vi "Get All Measured Values.vi"(0 "VISA Session In":refnum<visa-resource-name>="OXYMAT", 1 "Target Address":u8=16 format="%.0x", 2 "Source Address":u8=208 format="%.0x", 7 "Use Broadcast?(F)":bool, 11 "error in (no error)":errorcluster) -> (4 "VISA Session Out":refnum<visa-resource-name>, 6 "Message Header":T3 {"Source Address" format="%.0x"; "Target Address" format="%.0x"}, 8 "Measurements":cluster{"Measured value":dbl, "Dimension":T1}[](array[cluster]) {"Measured value" format="%#_6f"}, 10 "Measured variables":T2[](array[typedef]), 13 "Success":bool, 15 "error out":errorcluster)   [LabVIEW 2020, in "Siemens ELAN.lvlib"]
doc: "Using the Siemens ELAN protocol, gets all measured values from a channel. The input boolean 'Use Broadcast?' determines whether the values are actively requested, or whether this VI passively waits for a broadcast telegram. Returns array of measured real values and units of measure, plus a matching array of measured variable types. Also returns a boolean indicating that the addressed device provided a valid response.\n\n$Revision:: 0 $\n$Modtime:: yy-mm-dd hh:mm $\n$Author:: Dboyd $"
uses:
  Siemens ELAN.lvlib
  Unit Dimensions.ctl
  Measured variables.ctl
  Message Header.ctl
  Channel Status.ctl
panel:
  in  "Measured variable":T2
  in  "Dimension":T1
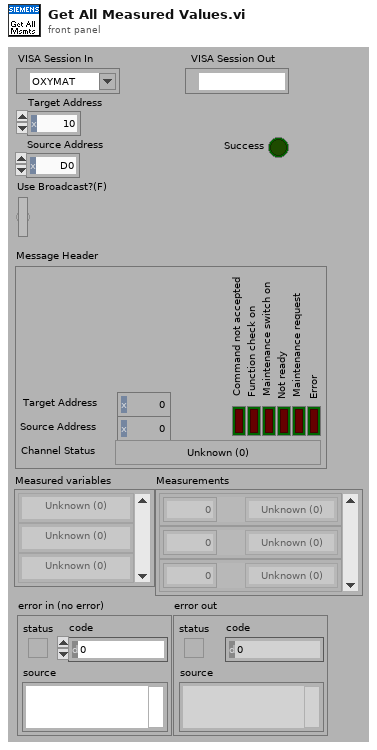
[diagram p1: front panel]
types:
  T1 = typedef "Siemens ELAN.lvlib/Unit Dimensions.ctl" = enum8{"Unknown (0)", "Pure number", "ppm", "ppb", "vpm", "vpm C1", "vpm C3", "vpm C6", "mg C/m^3", "mg/m^3", "%", "% v/v", "% of range", "% saturation", "%/°C", "%/K", "% w/w", "mV/pH", "mV/mbar", "nA/mbar", "S/m", "S/cm", "mS/m", "mS/cm", "uS/m", "uS/cm", "s", "min", "hr", "pA", "mA", "uV", "mV", "V", "mbar", "hPa", "ml/min", "kohm", "MOhm", "S", "°C", "Hz", "pH", "ug/l", "mg/l", "l/min", "uA", "mg/dm^3", "kPa", "kohm*cm", "MOhm*cm", "°", "Unknown (>51)"}
  T2 = typedef "Siemens ELAN.lvlib/Measured variables.ctl" = enum8{"Unknown (0)", "No component", "CO", "CO2", "CH4", "C6H14", "SO2", "NO", "NO2", "CHClF2 (R22)", "C3H8", "C4H10", "O2", "C5H12", "HC", "Pressure", "pH", "Temperature", "C2H4", "C2H2", "C3H6", "C4H6", "C4H8", "C2H6", "NH3", "N2O", "C6H6", "SF6", "CH3OH", "C2H5OH", "CH2Cl2", "C2H4Cl2", "CH3Cl", "C2H4O", "H2O (vapor)", "G/l", "Unknown (36)", "Unknown (37)", "Unknown (38)", "Unknown (39)", "Unknown (40)", "Unknown (41)", "Unknown (42)", "Unknown (43)", "Unknown (44)", "Unknown (45)", "Unknown (46)", "Unknown (47)", "Unknown (48)", "Unknown (49)", "Unknown (50)", "Unknown (51)", "Unknown (52)", "Unknown (53)", "Unknown (54)", "Unknown (55)", "Unknown (56)", "Unknown (57)", "Unknown (58)", "Unknown (59)", "Unknown (60)", "Unknown (61)", "Unknown (62)", "Unknown (63)", "Unknown (64)", "Unknown (65)", "Unknown (66)", "Unknown (67)", "Unknown (68)", "Unknown (69)", "Unknown (70)", "Unknown (71)", "Unknown (72)", "Unknown (73)", "Unknown (74)", "Unknown (75)", "Unknown (76)", "Unknown (77)", "Unknown (78)", "Unknown (79)", "Unknown (80)", "Unknown (81)", "Unknown (82)", "Unknown (83)", "Unknown (84)", "Unknown (85)", "Unknown (86)", "Unknown (87)", "Unknown (88)", "Unknown (89)", "Unknown (90)", "Unknown (91)", "Unknown (92)", "Unknown (93)", "Unknown (94)", "Unknown (95)", "Unknown ((96)", "Unknown (97)", "Unknown (98)", "Unknown (99)", "Ambient Pressure", "Unknown (>100)"}
  T3 = typedef "Siemens ELAN.lvlib/Message Header.ctl" = cluster{"Target Address":u8, "Source Address":u8, "Error":bool, "Maintenance request":bool, "Not ready":bool, "Maintenance switch on":bool, "Function check on":bool, "Command not accepted":bool, "Channel Status":T4}
  T4 = typedef "Siemens ELAN.lvlib/Channel Status.ctl" = enum8{"Unknown (0)", "Warm-up", "Pause", "Standby", "Measure", "Zero calibration", "Adjust component slope", "Unknown (7)", "Adjust curve dip", "Adjust linearization sensitivity", "Adjust temperature compensation", "Adjust pressure compensation", "Adjust linearization zero", "Adjust flow sensor", "Autocal", "Adjust phase", "Zero calibration of O2 sensor", "Synchronous zero calibration", "Purging for synchronous zero calibration", "Adjust analog output", "Adjust analog input", "Cleaning", "Unknown (>21)"}
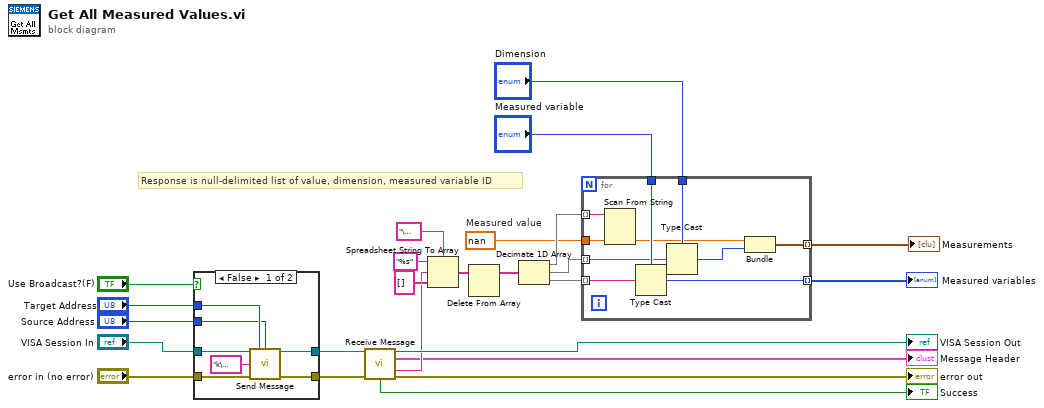
[diagram p0: block diagram]
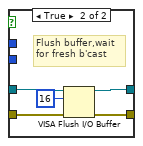
[diagram p2: hidden frame]
diagram:
  w5 = nan  # Measured value
  # "Response is null-delimited list of value, dimension, measured variable ID"
  n1 = case shown="False" "Use Broadcast?(F)" {
    tunnel: [w32 w36] -> w25
    tunnel: [w31 w34] -> w24
    tunnel: "VISA Session In" -> [w30 w37]
    tunnel: "error in (no error)" -> [w29 w35]
    tunnel: "Target Address" -> [w28 _]
    tunnel: "Source Address" -> [w27 _]
    frame False {
      n2 = call "Send Message.vi"("VISA Session In"=w30, "Target Address"=w28, "Source Address"=w27, "Command"="k\u0002", "error in (no error)"=w29) -> ("VISA Session Out"=w32:refnum<visa-resource-name>, "error out"=w31:errorcluster)  [unwired: 8 in, 1 out]
    }
    frame True {
      # "Flush buffer,wait\nfor fresh b'cast"
      n3 = VISA Flush I/O Buffer(VISA resource name=w37, mask (16)=u16 16, error in (no error)=w35) -> (VISA resource name out=w36:refnum<visa-resource-name>, error out=w34:errorcluster)
    }
  }
  n4 = call "Receive Message.vi"("VISA Session In"=w25, "error in (no error)"=w24) -> ("VISA Session Out"=→"VISA Session Out":refnum<visa-resource-name>, "Message Header"=→"Message Header":T3, "Response"=w15:string, "Success"=→"Success":bool, "error out"=→"error out":errorcluster)  [unwired: 8 in, 1 out]
  n5 = Spreadsheet String To Array(delimiter (Tab)="\u0000", format string="%s", spreadsheet string=w15, array type (2D Dbl)=string[] []) -> (array=w12:string[])
  n6 = Delete From Array(array=w12) -> (array with subset deleted=w11:string[])  [unwired: 2 in, 1 out]
  n7 = Decimate 1D Array(w11) -> (w6:string[], w9:string[], w10:string[])
  n8 = for {
    tunnel: "Dimension" -> [w47]
    tunnel: w10 -> [w42] mode=indexing
    tunnel: w9 -> [w41] mode=indexing
    tunnel: "Measured variable" -> [w46]
    tunnel: [w45] -> w4 mode=indexing
    tunnel: w6 -> [w44] mode=indexing
    tunnel: w5 -> [w43]
    tunnel: [w38] -> w2 mode=indexing
    n9 = Scan From String(input string=w44, default 1=w43) -> (output 1=w40:dbl)  [unwired: 3 in, 3 out]
    n10 = Type Cast(type=w46, x=w42) -> (*(type *) &x=w45:T2)
    n11 = Type Cast(type=w47, x=w41) -> (*(type *) &x=w39:T1)
    n12 = Bundle("Measured value"=w40, "Dimension"=w39) -> (w38:cluster{"Measured value":dbl, "Dimension":T1})  [unwired: 1 in]
  }
  "Measured variables" <- w4
  "Measurements" <- w2
